vi "NanonisProperties_raw.vi"(0 "Application ref in":refnum<vi>, 5 "Position (nm)":cluster{"X":dbl, "Z":dbl, "Y":dbl}, 11 "error in (no error)":errorcluster, 12 "Z Write?":bool) -> (4 "Application ref out":refnum<vi>, 8 "Current (pA)":sgl format="%#_6p", 15 "error out":errorcluster)   [LabVIEW 2017]
uses:
  <userlib>/Nanonis Prog Interface V5/Nanonis Prog Interface.lvlib
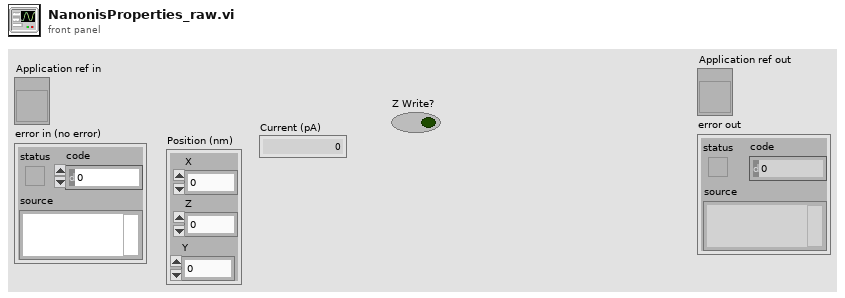
[diagram p1: front panel]
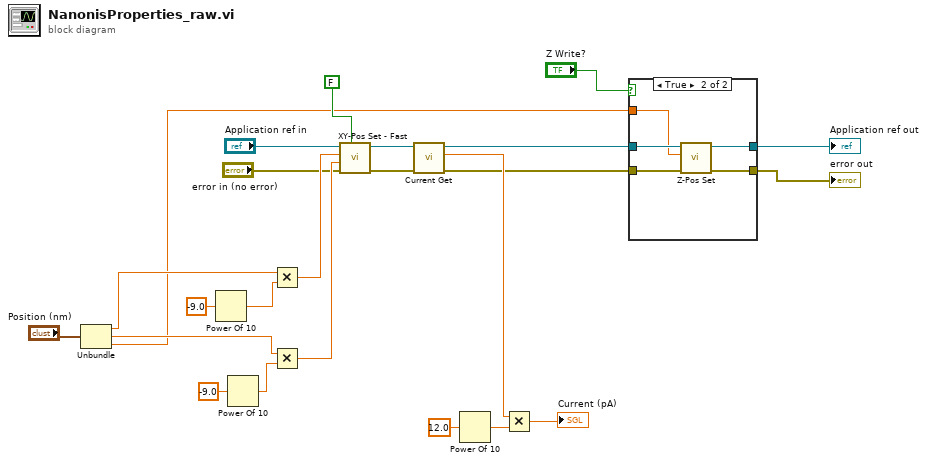
[diagram p0: block diagram]
diagram:
  n1 = Unbundle("Position (nm)") -> ("X"=w5:dbl, "Z"=w4:dbl, "Y"=w3:dbl)
  n2 = Power Of 10(x=-9.0) -> (10^x=w23:dbl)
  n3 = Power Of 10(x=-9.0) -> (10^x=w21:dbl)
  n4 = Multiply(x=w5, y=w23) -> (x*y=w19:dbl)
  n5 = Multiply(x=w4, y=w21) -> (x*y=w18:dbl)
  n6 = call <userlib>:"XY-Pos Set - Fast.vi"("Wait end-of-motion (T=True)"=FALSE, "error in (no error)"="error in (no error)", "Y (m)"=w18, "X (m)"=w19, "Application ref in"="Application ref in") -> ("error out"=w9:errorcluster, "Application ref out"=w10:refnum<vi>)  [unwired: 4 in]
  n7 = call <userlib>:"Current Get.vi"("Error in (no error)"=w9, "Application ref in"=w10) -> ("Error out"=w2:errorcluster, "Current (A)"=w14:sgl, "Application ref out"=w1:refnum<vi>)  [unwired: 5 in]
  n8 = Power Of 10(x=12.0) -> (10^x=w15:dbl)
  n9 = Multiply(x=w14, y=w15) -> (x*y=→"Current (pA)":dbl)
  n10 = case shown="True" "Z Write?" {
    tunnel: w1 -> [w26 w31]
    tunnel: w2 -> [w25 w30]
    tunnel: [w26 w29] -> w13
    tunnel: [w25 w28] -> w12
    tunnel: w3 -> [_ w27]
    frame False {
    }
    frame True {
      n11 = call <userlib>:"Z-Pos Set.vi"("error in (no error)"=w30, "Z position (m)"=w27, "Application ref in"=w31) -> ("error out"=w28:errorcluster, "Application ref out"=w29:refnum<vi>)  [unwired: 7 in]
    }
  }
  "Application ref out" <- w13
  "error out" <- w12
